vi "tcs shm cancel Callback command start LV.vi"(8 "error in (no error)":errorcluster) -> (0 "error out":errorcluster, 3 "function return":i32)   [LabVIEW 2016, in "SALLV_tcs.lvlib"]
doc: "int tcs_shm_cancelCallback_command_startLV();"
uses:
  SALLV_tcs.lvlib
  SALLV_tcs.so
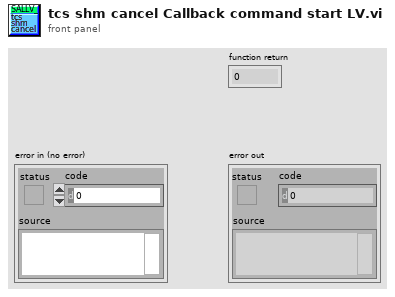
[diagram p1: front panel]
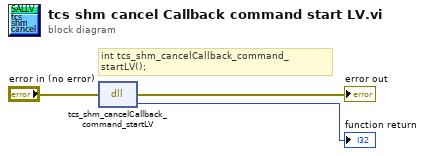
[diagram p0: block diagram]
diagram:
  # "int tcs_shm_cancelCallback_command_startLV();"
  n1 = dll-call lib="home/plotz/SALLV_tcs/SALLV_tcs.*" fn="tcs_shm_cancelCallback_command_startLV"(error in="error in (no error)") -> (error out=→"error out":errorcluster, →"function return":i32)  [unwired: 2 in, 1 out]
